vi "Periodic Tasks.vi"(8 "error in":errorcluster) -> ()   [LabVIEW 2016]
doc: "This VI runs in parallel to other tasks. It can contain as many user-defined periodic loops as you need. These can carry out PID or other sorts of timed response."
uses:
  <vilib>/Rock Robotics/WPI/Utilities/WPI_GetSetVariantRefNum.vi
  <vilib>/Rock Robotics/Network Tables/NT Read Number.vi
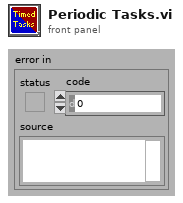
[diagram p1: front panel]
types:
  T1 = typedef "WPI_ServoDeviceRef.ctl" = cluster{"DeviceStatus":errorcluster, "PWM Channel":T2, "DeadBand":T3}
  T2 = typedef "FPGA_DIOPWMChannel.ctl" = enum8{"PWM 0", "PWM 1", "PWM 2", "PWM 3", "PWM 4", "PWM 5", "PWM 6", "PWM 7", "PWM 8", "PWM 9", "PWM MXP 0", "PWM MXP 1", "PWM MXP 2", "PWM MXP 3", "PWM MXP 4", "PWM MXP 5", "PWM MXP 6", "PWM MXP 7", "PWM MXP 8", "PWM MXP 9", "Invalid"}
  T3 = typedef "WPI_PWMDeadband.ctl" = cluster{"Name":string, "maxPositivePwm":i32, "minPositivePwm":i32, "centerPwm":i32, "maxNegativePwm":i32, "minNegativePwm":i32, "angularRange":u16}
  T4 = typedef "WPI_JoystickDevRef.ctl" = cluster{"Device":T5}
  T5 = typedef "WPI_JoystickDeviceEnum.ctl" = enum16{"USB 0", "USB 1", "USB 2", "USB 3", "USB 4", "USB 5"}
  T6 = typedef "WPI_MotorControlDeviceRef.ctl" = cluster{"DeviceStatus":errorcluster, "Type":T7, "PWM":cluster{"PWM Channel":T2, "DeadBand":T3}, "CAN":cluster{"Device Number":u8, "SetOutput VI Ref":variant, "GetOutput VI Ref":variant, "Enable VI Ref":variant, "Disable VI Ref":variant, "Data":variant}, "Invert":bool}
  T7 = typedef "WPI_MotorControlType.ctl" = enum16{"PWM", "CAN"}
  T8 = typedef "WPI_CANTalonSRX_GlobalStatus.ctl" = cluster{"Applied Throttle":dbl, "Module Enabled":bool, "CAN Error":errorcluster, "Closed Loop Error":dbl, "Forward Limit Switch Closed":bool, "Reverse Limit Switch Closed":bool, "Sensor Position":dbl, "Sensor Velocity":dbl, "Current":dbl, "Sticky Fault - Over Temp":bool, "Sticky Fault - Under Voltage":bool, "Sticky Fault - Forward Limit":bool, "Sticky Fault - Reverse Limit":bool, "Sticky Fault - Forward Soft Limit":bool, "Sticky Fault - Reverse Soft Limit":bool, "Brake is Enabled":bool, "Encoder Position":dbl, "Encoder Velocity":dbl, "Encoder Index Count":dbl, "Encoder A Pin State":bool, "Encoder B Pin State":bool, "Encoder Index Pin State":bool, "Analog In":dbl, "Analog In Velocity":dbl, "Temperature (C)":dbl, "Battery Voltage":dbl, "Control 5 Is Supported":bool, "Current Profile Slot Select":dbl, "Pos Div 8":bool, "Vel Div 4":bool, "Pulse Width Position":i32, "Pulse Width Velocity":i32, "Pulse Width Rise To Rise (us)":i32, "Pulse Width Rise To Fall (us)":i32, "Mot Prof Active Is Under Run":bool, "Mot Prof Active Has Under Run":bool, "Mot Prof Active Is Last":bool, "Mot Prof Active Velocity Only":bool, "Mot Prof Active Is Valid":bool, "Mot Prof Buffer Is Full":bool, "Mot Prof Active Profile Slot Select":i32, "Mot Prof NextID":i32, "Mot Prof Count":i32, "Mot Prof Active Velocity":dbl, "Mot Prof Active Position":dbl, "Mot Prof Output Enable":i32}
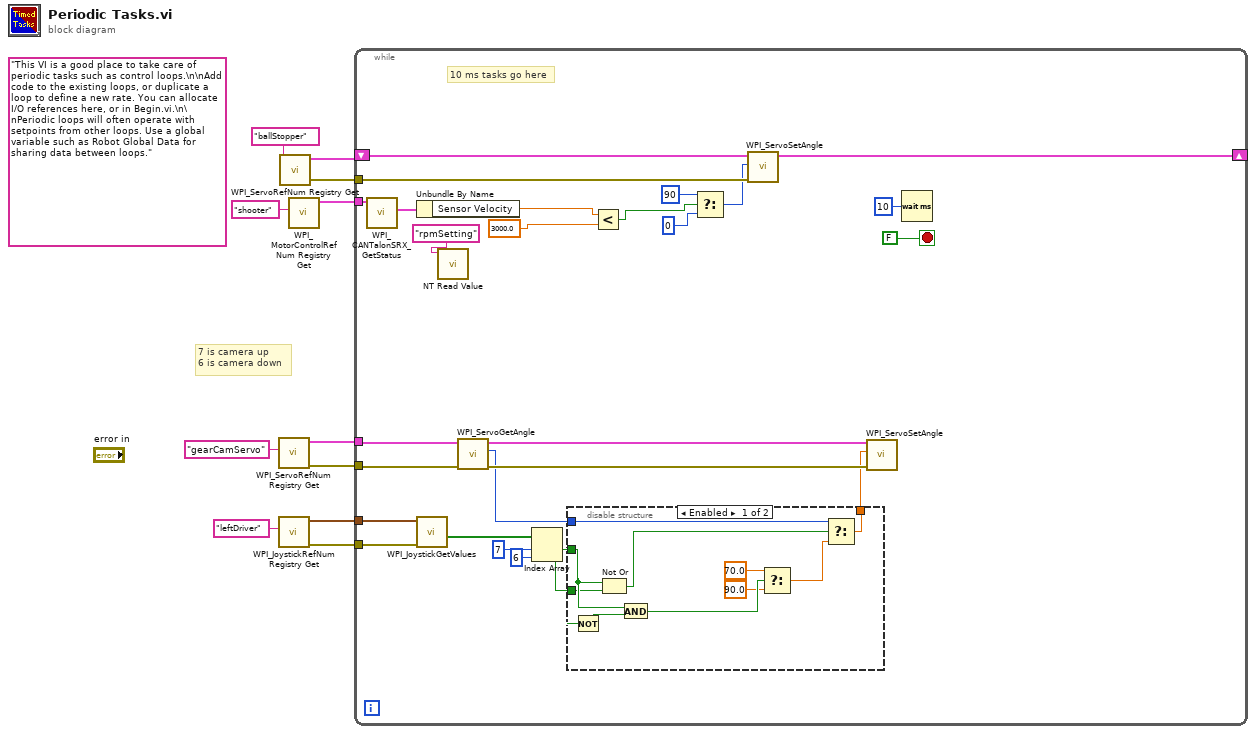
[diagram p0: block diagram]
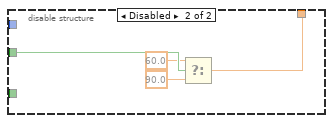
[diagram p2: hidden frame]
diagram:
  (unwired) "This VI is a good place to take care of periodic tasks such as control loops.\n\nAdd code to the existing loops, or duplicate a loop to define a new rate. You can allocate I/O references here, or in Begin.vi.\n\nPeriodic loops will often operate with setpoints from other loops. Use a global variable such as Robot Global Data for sharing data between loops."
  # "7 is camera up\n6 is camera down"
  n1 = call <vilib>:"WPI_ServoRefNum Registry Get.vi"("refnum name"="gearCamServo") -> ("error out"=w4:errorcluster, "ServoDeviceRef"=w5:T1)  [unwired: 9 in]
  n2 = call <vilib>:"WPI_JoystickRefNum Registry Get.vi"("refnum name"="leftDriver") -> ("error out"=w1:errorcluster, "JoystickDevRef"=w2:T4)  [unwired: 9 in]
  n3 = call <vilib>:"WPI_ServoRefNum Registry Get.vi"("refnum name"="ballStopper") -> ("error out"=w10:errorcluster, "ServoDeviceRef"=w11:T1)  [unwired: 9 in]
  n4 = call <vilib>:"WPI_MotorControlRefNum Registry Get.vi"("refnum name"="shooter") -> ("MotorControlDevRef"=w8:T6)  [unwired: 9 in, 1 out]
  n5 = while {
    tunnel: w10 -> [w35]
    tunnel: w8 -> [w30]
    shift-right: [w28] -> _
    shift-left: w11 -> [w36]
    tunnel: w5 -> [w23]
    tunnel: w4 -> [w22]
    tunnel: w2 -> [w26]
    tunnel: w1 -> [w25]
    stop <- FALSE stop-if-true
    # "10 ms tasks go here"
    n6 = call <vilib>:"WPI_CANTalonSRX_GetStatus.vi"("CAN Talon SRX Ref"=w30) -> ("Talon SRX Status"=w31:T8)  [unwired: 8 in, 2 out]
    n7 = Unbundle By Name(w31) -> ("Sensor Velocity"=w13:dbl)
    n8 = call <vilib>:"WPI_JoystickGetValues.vi"("error in (no error)"=w25, "JoystickDevRef"=w26) -> ("Buttons"=w24:bool[])  [unwired: 5 in, 4 out]
    n9 = call-poly <vilib>:"NT Read Value.vi"("Name"="rpmSetting") -> ()  [unwired: 9 in, 2 out]
    n10 = call <vilib>:"WPI_ServoGetAngle.vi"("ServoDeviceRef"=w23, "error in (no error)"=w22) -> ("ServoDeviceRef"=w21:T1, "Angle"=w19:u16, "error out"=w20:errorcluster)  [unwired: 6 in]
    n11 = Index Array(array=w24, index #1=7 ("index"), index #2=6 ("index")) -> (element #1=w18:bool, element #2=w15:bool)
    n12 = disable-structure shown="Enabled" {
      disable-tunnel: w19 -> [w48 _]
      disable-tunnel: w18 -> [w47 w51]
      disable-tunnel: [w46 w52] -> w17
      disable-tunnel: w15 -> [w45 _]
      frame Enabled {
        n13 = Not(x=w45) -> (.not. x?=w43:bool)
        n14 = Not Or(1:w45, 2:w47) -> (0:w39:bool)
        n15 = And(x=w47, y=w43) -> (x .and. y?=w42:bool)
        n16 = Select(t=70.0, s=w42, f=90.0) -> (s? t:f=w44:dbl)
        n17 = Select(t=w48, s=w39, f=w44) -> (s? t:f=w46:dbl)
      }
      frame Disabled {
        n18 = Select(t=60.0, s=w51, f=90.0) -> (s? t:f=w52:dbl)
      }
    }
    n19 = Less?(x=w13, y=3000.0 ("x")) -> (x < y?=w14:bool)
    n20 = Select(t=90, s=w14, f=0) -> (s? t:f=w32:i32)
    n21 = call <vilib>:"WPI_ServoSetAngle.vi"("error in (no error)"=w35, "Angle"=w32, "ServoDeviceRef"=w36) -> ("ServoDeviceRef"=w28:T1)  [unwired: 7 in, 1 out]
    n22 = call <vilib>:"WPI_ServoSetAngle.vi"("error in (no error)"=w20, "Angle"=w17, "ServoDeviceRef"=w21) -> ()  [unwired: 7 in, 2 out]
    n23 = Wait (ms)(milliseconds to wait=u32 10) -> ()  [unwired: 1 out]
  }
